vi "Config File - Read Config File.vi"(7 "section names (all)":string[](array[string]), 8 "error in (no error)":errorcluster, 9 "default values":map{string, map{string, string}}(c390), 11 "config file path":path) -> (0 "error out":errorcluster, 1 "config settings":map{string, map{string, string}}(c390))   [LabVIEW 2019]
doc: "<b>Description</b> Read a configuration (.ini) file into a string-typed map. Use the <b>Get From Map As Type.vim</b> to read keys from sections. The underlying implementation of the file reader is based on the stock Configuration File VIs.\n\n<b>Inputs</b>\n<b>default values</b>: A map containing default sections and values.\n<b>config file path</b>: Path of input config file to read.\n<b>section names</b>: A list of section names to read. Default behavior is to read all sections. \n\n<b>Outputs</b>\n<b>config settings</b>: Content of the config file. All values are represented as raw strings.\n\nBSD 3-Clause License\n\nCopyright (c) 2021, TauTerra, LLC\nAll rights reserved.\n\nRedistribution and use in source and binary forms, with or without\nmodification, are permitted provided that the following conditions are met:\n\n1. Redistributions of source code must retain the above copyright notice, this\n list of conditions and the following disclaimer.\n\n2. Redistributions in binary form must reproduce the above copyright notice,\n this list of conditions and the following disclaimer in the documentation\n and/or other materials provided with the distribution.\n\n3. Neither the name of the copyright holder nor the names of its\n contributors may be used to endorse or promote products derived from\n this software without specific prior written permission.\n\nTHIS SOFTWARE IS PROVIDED BY THE COPYRIGHT HOLDERS AND CONTRIBUTORS \"AS IS\"\nAND ANY EXPRESS OR IMPLIED WARRANTIES, INCLUDING, BUT NOT LIMITED TO, THE\nIMPLIED WARRANTIES OF MERCHANTABILITY AND FITNESS FOR A PARTICULAR PURPOSE ARE\nDISCLAIMED. IN NO EVENT SHALL THE COPYRIGHT HOLDER OR CONTRIBUTORS BE LIABLE\nFOR ANY DIRECT, INDIRECT, INCIDENTAL, SPECIAL, EXEMPLARY, OR CONSEQUENTIAL\nDAMAGES (INCLUDING, BUT NOT LIMITED TO, PROCUREMENT OF SUBSTITUTE GOODS OR\nSERVICES; LOSS OF USE, DATA, OR PROFITS; OR BUSINESS INTERRUPTION) HOWEVER\nCAUSED AND ON ANY THEORY OF LIABILITY, WHETHER IN CONTRACT, STRICT LIABILITY,\nOR TORT (INCLUDING NEGLIGENCE OR OTHERWISE) ARISING IN ANY WAY OUT OF THE USE\nOF THIS SOFTWARE, EVEN IF ADVISED OF THE POSSIBILITY OF SUCH DAMAGE."
uses:
  <vilib>/Utility/miscctls.llb/LVMapReplaceAction.ctl
  <vilib>/Utility/config.llb/Read Key (String).vi
  <vilib>/Utility/config.llb/NI_LVConfig.lvlib
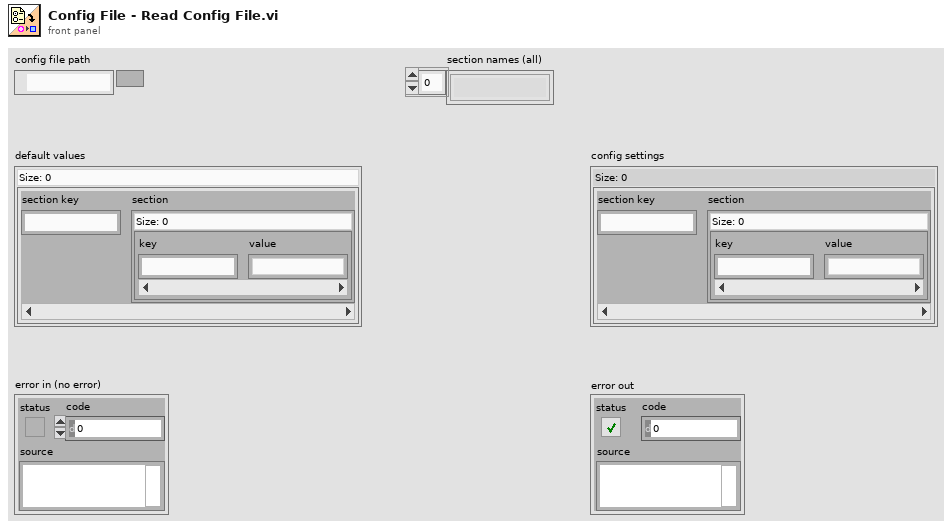
[diagram p1: front panel]
types:
  T1 = typedef "LVMapReplaceAction.ctl" = enum32{"Modify Entry only if found", "Add or Modify Entry", "Delete Entry"}
  T2 = typedef "NI_LVConfig.lvlib/Config Data RefNum.ctl" = refnum<k1>
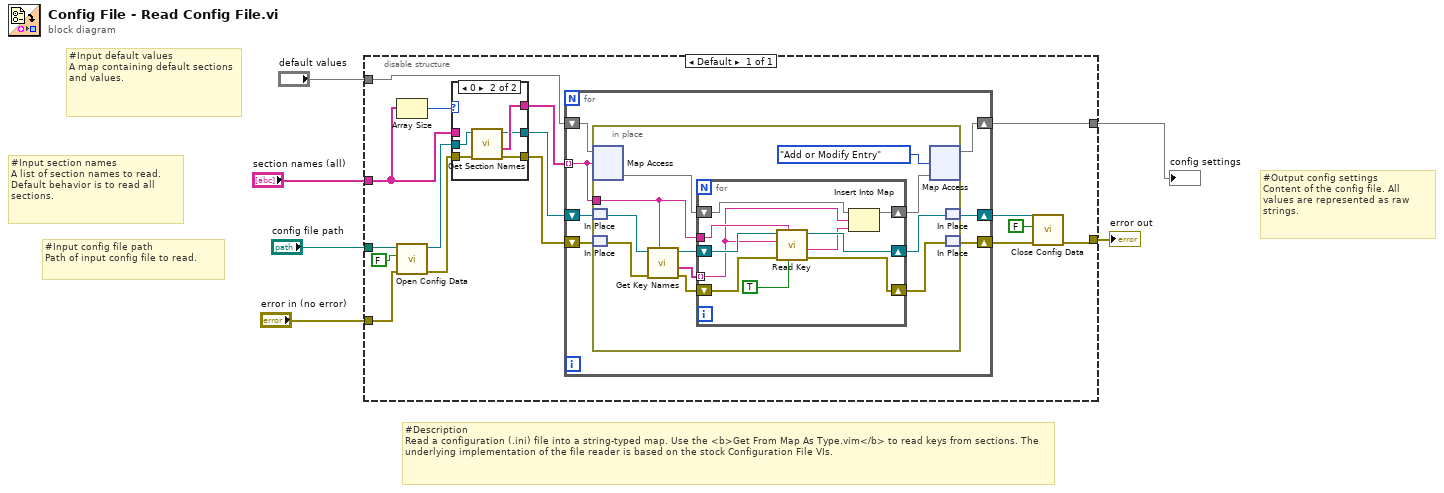
[diagram p0: block diagram]
diagram:
  # "#Output config settings\nContent of the config file. All values are represented as raw strings."
  # "#Input default values\nA map containing default sections and values."
  # "#Input config file path\nPath of input config file to read."
  # "#Input section names\nA list of section names to read. Default behavior is to read all sections."
  # "#Description\nRead a configuration (.ini) file into a string-typed map. Use the <b>Get From Map As Type.vim</b> to read keys from sections. The underlying implementation of the file reader is based on the stock Configuration File VIs."
  n1 = disable-structure shown="Default" {
    disable-tunnel: "config file path" -> [w22]
    disable-tunnel: "error in (no error)" -> [w21]
    disable-tunnel: "section names (all)" -> [w17]
    disable-tunnel: "default values" -> [w13]
    disable-tunnel: [w12] -> w2
    disable-tunnel: [w9] -> w1
    frame Enabled {
      n2 = Array Size(array=w17) -> (size(s)=w18:i32)
      n3 = call <vilib>:"Open Config Data.vi"("error in (no error)"=w21, "create file if necessary (T)"=FALSE, "configuration file path"=w22) -> ("error out"=w19:errorcluster, "refnum"=w20:T2)  [unwired: 6 in, 1 out]
      n4 = case shown="0" w18 {
        tunnel: w20 -> [w52 w58]
        tunnel: w19 -> [w51 w57]
        tunnel: [w53 w56] -> w14
        tunnel: w17 -> [w53 _]
        tunnel: [w52 w55] -> w16
        tunnel: [w51 w54] -> w15
        frame Default {
        }
        frame 0 {
          n5 = call <vilib>:"Get Section Names.vi"("error in (no error)"=w57, "refnum"=w58) -> ("error out"=w54:errorcluster, "section names"=w56:string[], "refnum out"=w55:T2)  [unwired: 7 in]
        }
      }
      n6 = for {
        shift-right: [w24] -> w11
        shift-left: w16 -> [w27]
        tunnel: w14 -> [w28] mode=indexing
        shift-right: [w25] -> w12
        shift-left: w13 -> [w29]
        shift-right: [w23] -> w10
        shift-left: w15 -> [w26]
        n7 = in-place {
          in-place-border: w28 -> [w40]
          n8 = in-place-map #1(w29, w28) -> (w37:map{string, string})  [unwired: 1 in, 1 out]
          n9 = in-place-match #2(w27) -> (w33:T2)
          n10 = in-place-match #3(w26) -> (w32:errorcluster)
          n11 = call <vilib>:"Get Key Names.vi"("section"=w40, "error in (no error)"=w32, "refnum"=w33) -> ("error out"=w34:errorcluster, "key names"=w38:string[], "refnum out"=w39:T2)  [unwired: 5 in, 1 out]
          n12 = for {
            tunnel: w40 -> [w50]
            tunnel: w38 -> [w45] mode=indexing
            shift-right: [w48] -> w30
            shift-left: w39 -> [w49]
            shift-right: [w43] -> w35
            shift-left: w37 -> [w46]
            shift-right: [w41] -> w31
            shift-left: w34 -> [w42]
            n13 = call-poly <vilib>:"Read Key.vi"("read raw string? (F)"=TRUE, "section"=w50, "error in (no error)"=w42, "key"=w45, "refnum"=w49) -> ("error out"=w41:errorcluster, "value"=w44:string, "refnum out"=w48:T2)  [unwired: 3 in, 1 out]
            n14 = Insert Into Map(map in=w46, key=w45, value=w44) -> (map out=w43:map{string, string})  [unwired: 2 out]
          }
          n15 = in-place-map #1(w35, LVMapReplaceAction."Add or Modify Entry" ("action")) -> (w25:map{string, map{string, string}})  [unwired: 2 out]
          n16 = in-place-match #2(w30) -> (w24:T2)
          n17 = in-place-match #3(w31) -> (w23:errorcluster)
        }
      }
      n18 = call <vilib>:"Close Config Data.vi"("error in (no error)"=w10, "write file if changed (T)"=FALSE, "refnum"=w11) -> ("error out"=w9:errorcluster)  [unwired: 7 in, 1 out]
    }
  }
  "config settings" <- w2
  "error out" <- w1
